vi "Create or Update Palette.vi"(8 "error in (no error)":errorcluster, 10 "Suggestions":cluster{"Class Name":string, "Count":i32}[](array[cluster]), 11 "VIAppRef":refnum<vi>) -> (0 "error out":errorcluster, 3 "reference out":refnum<vi>)   [LabVIEW 2024]
uses:
  <vilib>/Palette API/Palette Menu/Public Type Define/Item.ctl
  <vilib>/Palette API/Palette Menu/Public Type Define/Palette type.ctl
  <vilib>/Palette API/Palette Menu/Public Type Define/Palette Data.ctl
  <vilib>/Palette API/Palette Menu/Public Type Define/View Format.ctl
  <vilib>/Palette API/Palette Menu/Public Type Define/Items.ctl
  <vilib>/Palette API/Palette Menu/Public Type Define/Help Info.ctl
  <vilib>/Palette API/Palette Menu/Public Type Define/Synchronize Info.ctl
  <vilib>/Palette API/Palette Menu/Palette Menu.lvlib
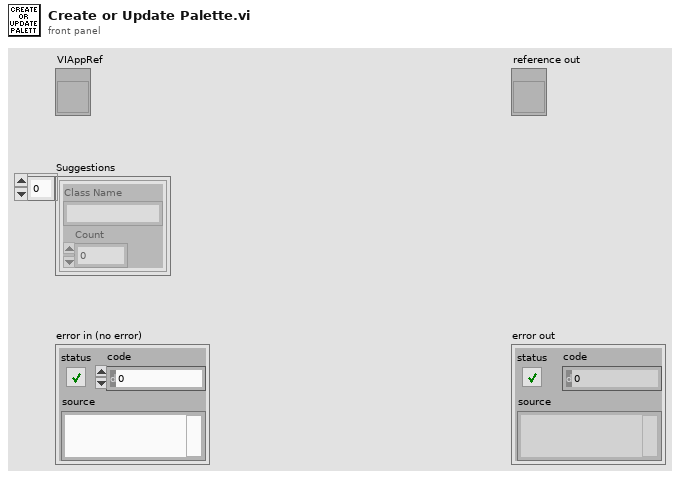
[diagram p1: front panel]
types:
  T1 = typedef "Palette Menu.lvlib/Palette type.ctl" = i32
  T2 = typedef "Palette Menu.lvlib/Item.ctl" = cluster{"item path":path, "library path":path, "use default lvlib palette":bool, "short name":string, "place VI contents":bool, "hide synchronized item":bool, "reserve spot for synch item":bool, "configure when placing VI contents":bool}
  T3 = typedef "Palette Menu.lvlib/Palette Data.ctl" = cluster{"display name":string, "view format":T4, "palette width":i16, "items":T5, "256 color icon":picture, "B&W color icon":picture, "help information":T6, "palette description":string, "synchronize information":T7}
  T4 = typedef "Palette Menu.lvlib/View Format.ctl" = u16
  T5 = typedef "Palette Menu.lvlib/Items.ctl" = T2[]
  T6 = typedef "Palette Menu.lvlib/Help Info.ctl" = cluster{"help tag":string, "help file path ":path}
  T7 = typedef "Palette Menu.lvlib/Synchronize Info.ctl" = cluster{"synchronize with directory":bool, "synchronize directory path":path}
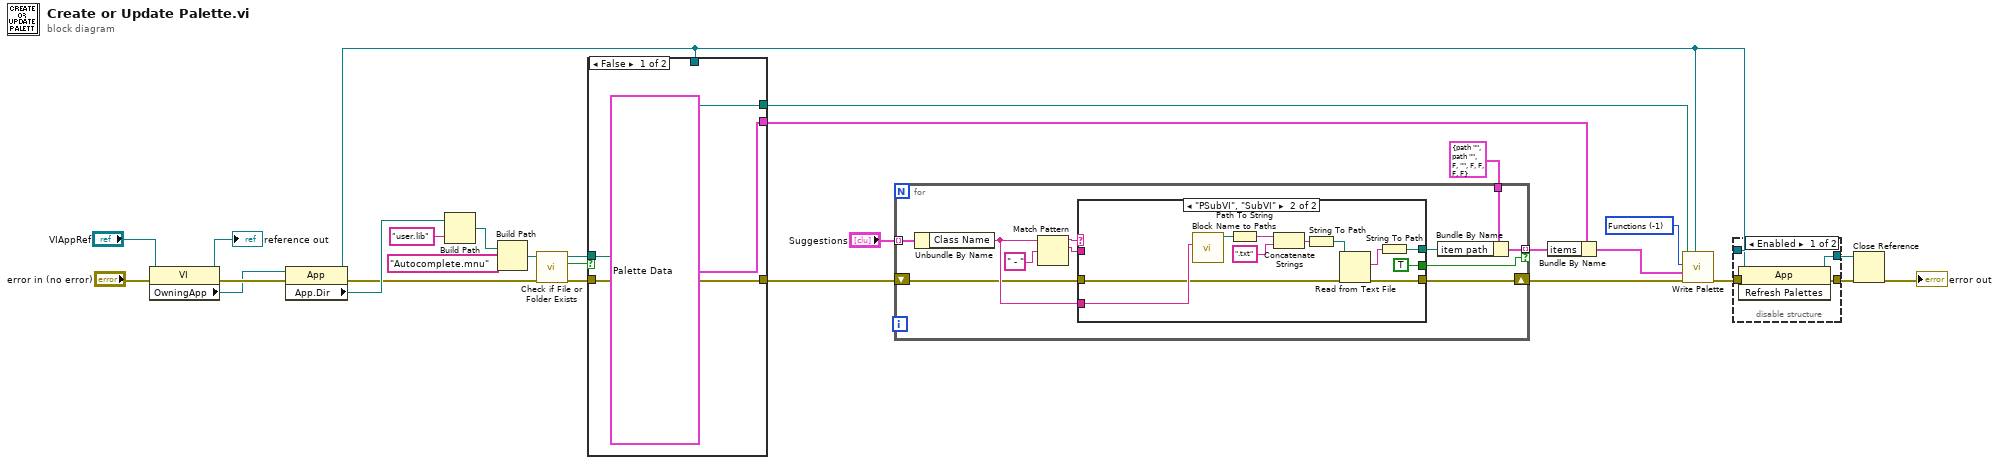
[diagram p0: block diagram]
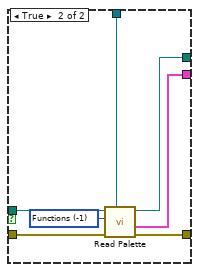
[diagram p4: hidden frame]
diagram:
  w17 = T1 -1 items=["Functions"=-1, "Controls"=-2] ("palette type")
  n1 = property class="VI"(reference="VIAppRef", error in="error in (no error)") -> (reference out=→"reference out":refnum<vi>, error out=w9:errorcluster, "OwningApp"=w7:refnum<vi>)
  n2 = property class="App"(reference=w7, error in=w9) -> (reference out=w12:refnum<vi>, error out=w13:errorcluster, "App.Dir"=w26:path)
  n3 = Build Path(base path=w26, name or relative path="user.lib") -> (appended path=w24:path)
  n4 = Build Path(base path=w24, name or relative path="Autocomplete.mnu") -> (appended path=w27:path)
  n5 = call <vilib>:"Check if File or Folder Exists.vi"("error in (no error)"=w13, "path"=w27) -> ("error out"=w23:errorcluster, "file or folder exists?"=w22:bool, "dup path"=w21:path)  [unwired: 7 in]
  n6 = case shown="False" w22 {
    tunnel: w23 -> [w30 w38]
    tunnel: w21 -> [w31 w37]
    tunnel: [w31 w35] -> w16
    tunnel: [T3 {"display name"="Autocomplete", "view format"=0, "palette width"=4, "items"=[], "256 color icon"=bytes[3232], "B&W color icon"=bytes[0], "help information"={"help tag"="", "help file path "=path ""}, "palette description"="", "synchronize information"={"synchronize with directory"=FALSE, "synchronize directory path"=path ""}} ("palette data") w34] -> w20
    tunnel: [w30 w33] -> w2
    tunnel: w12 -> [_ w32]
    frame False {
    }
    frame True {
      w36 = T1 -1 items=["Functions"=-1, "Controls"=-2] ("palette type")
      n7 = call <vilib>:"Read Palette.vi"("application reference"=w32, "error in (no error)"=w38, "palette type"=w36, "palette path"=w37) -> ("error out"=w33:errorcluster, "palette data"=w34:T3, "duplicate palette path"=w35:path)  [unwired: 5 in]
    }
  }
  n8 = for {
    tunnel: T2 {"item path"=path "", "library path"=path "", "use default lvlib palette"=FALSE, "short name"="", "place VI contents"=FALSE, "hide synchronized item"=FALSE, "reserve spot for synch item"=FALSE, "configure when placing VI contents"=FALSE} ("items") -> [w49]
    tunnel: [w48] -> w18 mode=indexing if=w44
    tunnel: "Suggestions" -> [w47] mode=indexing
    shift-right: [w39] -> w1
    shift-left: w2 -> [w40]
    n9 = Unbundle By Name(w47) -> ("Class Name"=w41:string)
    n10 = Match Pattern(string=w41, regular expression=" - " ("search string/char (-)")) -> (before substring=w45:string, match substring=w42:string)  [unwired: 1 in, 2 out]
    n11 = case shown="\"PSubVI\", \"SubVI\"" w45 {
      tunnel: [_ TRUE ("Boolean")] -> w44
      tunnel: [_ w54] -> w43
      tunnel: w42 -> [_ _]
      tunnel: w41 -> [_ w53]
      tunnel: w40 -> [w50 w52]
      tunnel: [w50 w51] -> w39
      frame Default {
      }
      frame "PSubVI", "SubVI" {
        n12 = call "Block Name to Paths.vi"("Block Name"=w53) -> ("Block Path"=w59:path)  [unwired: 9 in, 1 out]
        n13 = Path To String(path=w59) -> (string=w56:string)
        n14 = Concatenate Strings(w56, ".txt" ("string")) -> (w57:string)
        n15 = String To Path(string=w57) -> (path=w60:path)
        n16 = Read from Text File(file (use dialog)=w60, error in=w52) -> (text=w58:string, error out=w51:errorcluster)  [unwired: 2 in, 2 out]
        n17 = String To Path(string=w58) -> (path=w54:path)
      }
    }
    n18 = Bundle By Name(cluster=w49, "item path"=w43) -> (w48:T2)
  }
  n19 = Bundle By Name(cluster=w20, "items"=w18) -> (w15:T3)
  n20 = call <vilib>:"Write Palette.vi"("application reference"=w12, "error in (no error)"=w1, "palette data"=w15, "palette type"=w17, "palette path"=w16) -> ("error out"=w14:errorcluster)  [unwired: 6 in]
  n21 = disable-structure shown="Enabled" {
    disable-tunnel: w14 -> [w65 w67]
    disable-tunnel: w12 -> [w64 w66]
    disable-tunnel: [w63 w67] -> w6
    disable-tunnel: [w62 w66] -> w4
    frame Enabled {
      n22 = invoke class="App" method="Refresh Palettes"(reference=w64, error in=w65) -> (reference out=w62:refnum<vi>, error out=w63:errorcluster)  [unwired: 1 in, 1 out]
    }
    frame Disabled {
    }
  }
  n23 = Close Reference(reference=w4, error in (no error)=w6) -> (error out=→"error out":errorcluster)
